vi "Indent.vi"(8 "Indent":bool, 9 "Text.Selection Start":u32, 10 "Text.Selection End":u32, 11 "string in":string) -> (1 "indent string":string, 2 "New SelStart":i32, 3 "New SelEnd":i32)   [LabVIEW 2019]
uses:
  <vilib>/Utility/error.llb/whitespace.ctl
panel:
  out "# lines":i32
  out "line number start":i32
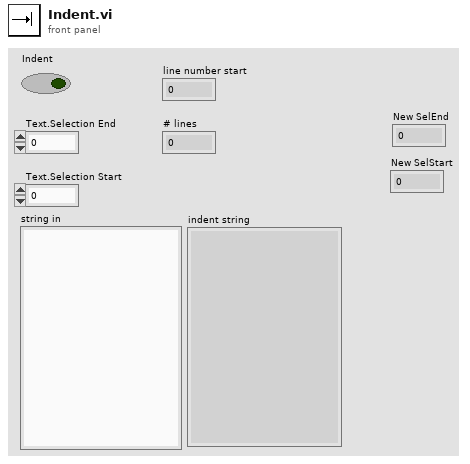
[diagram p1: front panel]
types:
  T1 = typedef "whitespace.ctl" = u16
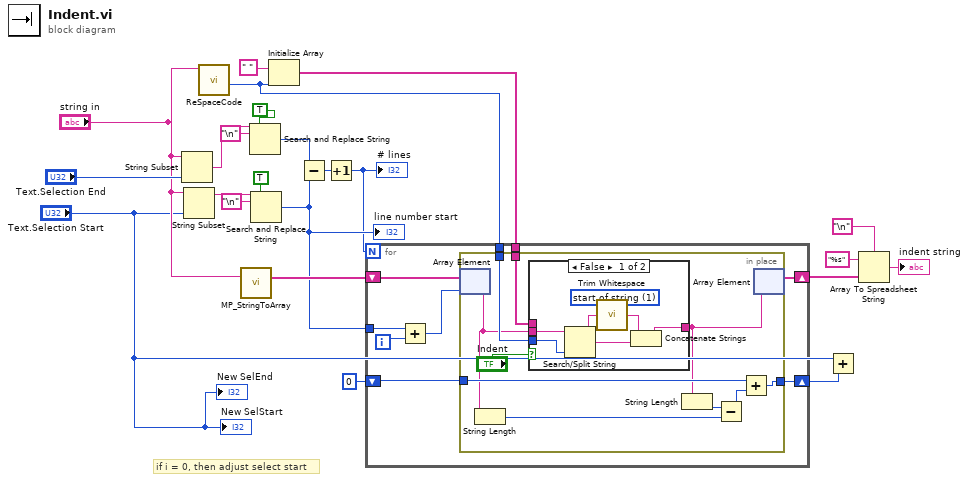
[diagram p0: block diagram]
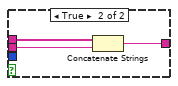
[diagram p2: hidden frame]
diagram:
  # "if i = 0, then adjust select start"
  n1 = String Subset(string="string in", length (rest)="Text.Selection End") -> (substring=w13:string)  [unwired: 1 in]
  n2 = String Subset(string="string in", length (rest)="Text.Selection Start") -> (substring=w9:string)  [unwired: 1 in]
  n3 = call <userlib>:"ReSpaceCode.vi"("Code"="string in") -> ("min value"=w5:i32)  [unwired: 9 in, 1 out]
  n4 = call <userlib>:"MP_StringToArray.vi"("write buffer"="string in") -> ("Array"=w16:string[])  [unwired: 10 in]
  n5 = Search and Replace String(replace all?=TRUE ("replace all? (F)"), input string=w13, search string="\n") -> (number of replacements=w14:i32)  [unwired: 5 in, 3 out]
  n6 = Search and Replace String(replace all?=TRUE ("replace all? (F)"), input string=w9, search string="\n") -> (number of replacements=w7:i32)  [unwired: 5 in, 3 out]
  "line number start" <- w7
  n7 = Initialize Array(" " ("search string"), w5) -> (w23:string[])
  n8 = Subtract(x=w14, y=w7) -> (x-y=w15:i32)
  n9 = Increment(x=w15) -> (x+1=w6:i32)
  "# lines" <- w6
  n10 = for {
    N: w6 -> [_]
    tunnel: w7 -> [w31]
    shift-right: [w28] -> w17
    shift-left: w16 -> [w30]
    tunnel: w23 -> [w27]
    tunnel: w5 -> [w26]
    shift-right: [w25] -> w3
    shift-left: 0 -> [w24]
    i -> [w32]
    n11 = Add(x=w31, y=w32) -> (x+y=w29:i32)
    n12 = in-place {
      in-place-border: w27 -> [w42]
      in-place-border: w26 -> [w40]
      in-place-border: [w39] -> w25
      in-place-border: w24 -> [w38]
      n13 = in-place-array #1(w30, w29) -> (w36:string)
      n14 = String Length(string=w36) -> (length=w33:i32)
      n15 = case shown="False" "Indent" {
        tunnel: [w43 w50] -> w37
        tunnel: w36 -> [w49 w52]
        tunnel: w42 -> [_ w51]
        tunnel: w40 -> [w48 _]
        frame False {
          w45 = T1 1 items=["both", "start of string", "end of string"] ("location (both)")
          n16 = Search/Split String(string=w49, offset (0)=w48) -> (substring before match=w47:string, match + rest of string=w46:string)  [unwired: 1 in, 1 out]
          n17 = call <vilib>:"Trim Whitespace.vi"("string"=w47, "location (both)"=w45) -> ("trimmed string"=w44:string)
          n18 = Concatenate Strings(w44, w46) -> (w43:string)
        }
        frame True {
          n19 = Concatenate Strings(w51, w52) -> (w50:string)
        }
      }
      n20 = String Length(string=w37) -> (length=w34:i32)
      n21 = Subtract(x=w34, y=w33) -> (x-y=w35:i32)
      n22 = Add(x=w38, y=w35) -> (x+y=w39:i32)
      n23 = in-place-array #1(w37) -> (w28:string[])  [unwired: 1 out]
    }
  }
  n24 = Add(x="Text.Selection Start", y=w3) -> ()  [unwired: 1 out]
  n25 = Array To Spreadsheet String(delimiter (Tab)="\n", array=w17, 3:"%s" ("format string")) -> (spreadsheet string=→"indent string":string)
  "New SelEnd" <- "Text.Selection Start"
  "New SelStart" <- "Text.Selection Start"
